vi "MasterStateController.vi"() -> (8 "Master State Out":T1(ring))   [LabVIEW 2020]
doc: "This is the master robot state controller. The master robot state can affect any of the subsystem state controllers."
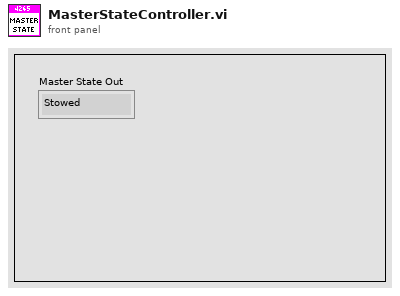
[diagram p1: front panel]
types:
  T1 = enum16{"Stowed", "Balancing", "Scoring", "Hoppering", "Ground", "Shelf"}
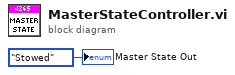
[diagram p0: block diagram]
diagram:
  "Master State Out" <- T1."Stowed" ("Master State Out")
